vi "FTW-JSON-Core-NumericType.vi"(1 "LabVIEW Type":T2) -> (0 "Scalar NumType":T1(ring))   [LabVIEW 2015]
uses:
  reflection/FTW-Reflection-Types.ctl
panel:
  # "Inputs"
  # "Outputs"
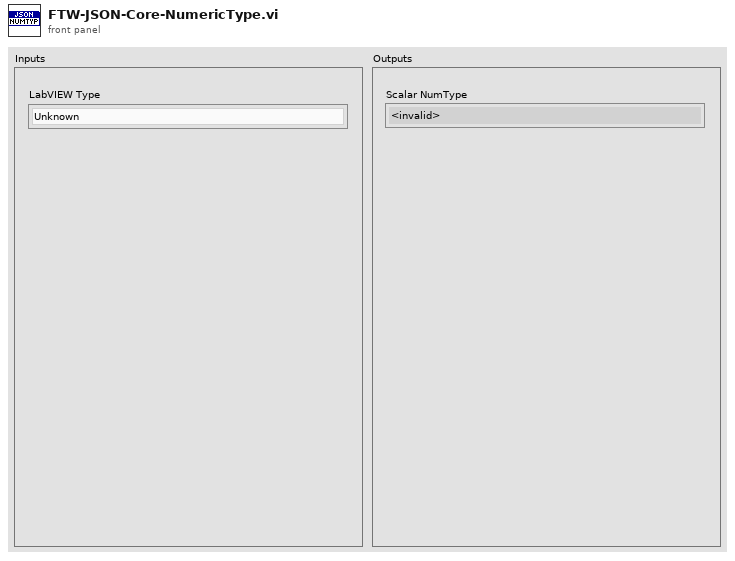
[diagram p1: front panel]
types:
  T1 = enum8{"<invalid>", "iB", "iW", "iL", "iQ", "uB", "uW", "uL", "uQ", "fS", "fD", "fX", "cS", "cD", "cX"}
  T2 = typedef "FTW-Reflection-Types.ctl" = enum16{"Unknown", "Void", "Array", "Cluster", "LVObject", "Boolean", "I8", "I16", "I32", "I64", "U8", "U16", "U32", "U64", "SGL", "DBL", "EXT", "CSG", "CDB", "CXT", "FXP", "EnumU8", "EnumU16", "EnumU32", "EnumU64", "SGLwithUnit", "DBLwithUnit", "EXTwithUnit", "CSGwithUnit", "CDBwithUnit", "CXTwithUnit", "String", "Path", "Picture", "Tag", "LVVariant", "Timestamp", "WaveformI8", "WaveformI16", "WaveformI32", "WaveformI64", "WaveformU8", "WaveformU16", "WaveformU32", "WaveformU64", "WaveformSGL", "WaveformDBL", "WaveformEXT", "WaveformCSG", "WaveformCDB", "WaveformCXT", "WaveformDigital", "WaveformUnknownType", "DigitalData", "DynamicData", "ExternalData", "FileByteStream", "TDMStream", "dotNET", "ActiveX", "VIServerReference", "VIReference", "ApplicationInstance", "Menu", "ConnectionDataSocket", "ConnectionVISA", "ConnectionBluetooth", "ConnectionIrDA", "ConnectionTCP", "ConnectionUDP", "ConnectionHTTPClient", "ConnectionFTP", "Occurrence", "Notifier", "Queue", "Rendezvous", "Semaphore", "RTFIFO", "EventPublisher", "EventRegistration", "EventCallback", "DataValueReference", "GenericClass", "GenericClassTag", "GenericClassDeepCopy", "GenericClassFlattened", "GenericClassTagFlattened", "GenericReferenceType", "WindowsRegistry", "OverloadedDatalogRef", "ReferenceUnknownType", "ByteArray", "ConPaneInterface", "FTWObject"}
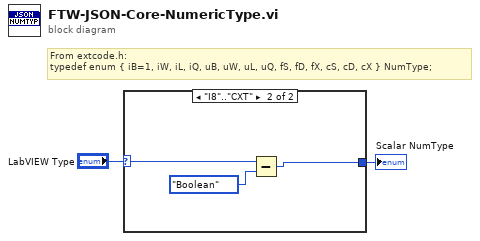
[diagram p0: block diagram]
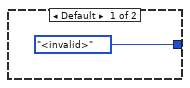
[diagram p2: hidden frame]
diagram:
  # "From extcode.h:\ntypedef enum {\tiB=1, iW, iL, iQ, uB, uW, uL, uQ, fS, fD, fX, cS, cD, cX } NumType;"
  n1 = case shown="\"I8\"..\"CXT\"" "LabVIEW Type" {
    selector: "LabVIEW Type" -> [_ w6]
    tunnel: [T1."<invalid>" ("Scalar NumType") w4] -> w1
    frame Default {
    }
    frame "I8".."CXT" {
      n2 = Subtract(x=w6, y=FTW-Reflection-Types."Boolean" ("LabVIEW Type")) -> (x-y=w4:u16)
    }
  }
  "Scalar NumType" <- w1
